vi "read pair information.vi"(8 "error in":errorcluster, 11 "UDP Broadcast Editor Node in":refnum<class "TEC editor node.lvclass">) -> (0 "error out":errorcluster, 2 "pair info":T1, 3 "UDP Broadcast Editor Node out":refnum<class "TEC editor node.lvclass">)   [LabVIEW 2014, in "TEC editor node.lvclass"]
uses:
  TEC editor node.lvclass
  pair information.ctl
  TEC editor node.lvclass/TEC editor node.ctl
  <vilib>/NI/Configuration Framework/serializable configuration/NISE_CEF_serializable configuration.lvclass
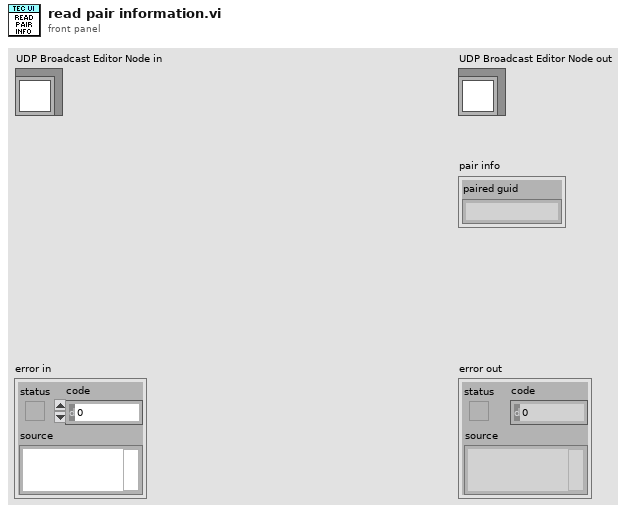
[diagram p1: front panel]
types:
  T1 = typedef "TEC editor node.lvclass/pair information.ctl" = cluster{"paired guid":string}
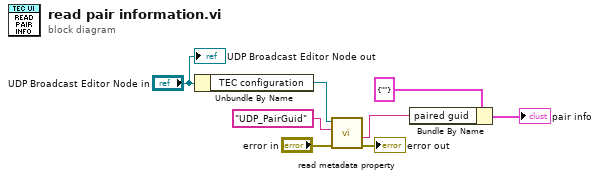
[diagram p0: block diagram]
diagram:
  n1 = Unbundle By Name("UDP Broadcast Editor Node in") -> ("TEC configuration"=w7:refnum<class "TEC configuration.lvclass">)
  n2 = call <vilib>:"read metadata property.vi"("error in"="error in", "key"="UDP_PairGuid", "configuration in"=w7) -> ("error out"=→"error out":errorcluster, "value"=w1:string)  [unwired: 5 in, 2 out]
  n3 = Bundle By Name(cluster=T1 {"paired guid"=""} ("pair info"), "paired guid"=w1) -> (→"pair info":T1)
  "UDP Broadcast Editor Node out" <- "UDP Broadcast Editor Node in"
